vi "IO输出界面.vi"(8 "错误输入（无错误）":errorcluster, 10 "界面切换队列":refnum<queue>, 11 "VISA资源名称输入":refnum<visa-resource-name>) -> (0 "错误输出":errorcluster, 3 "VISA资源名称输出":refnum<visa-resource-name>)   [LabVIEW 2018]
panel:
  out "毫秒计时值":u32
  in  "枚举":T1(ring)
  in  "选项卡控件":enum32{"选项卡 1", "选项卡 2"}(tab)
  out "无":bool
  out "无":bool
  out "无":bool
  out "无":bool
  out "无":bool
  out "无":bool
  out "Y30D-11#启动":bool
  out "Y30E-13#启动":bool
  out "Y30F-15#启动":bool
  out "Y100-2#启动":bool
  out "Y101-4#启动":bool
  out "Y102-6#启动":bool
  out "Y103-8#启动":bool
  out "Y104-10#启动":bool
  out "Y105-12#启动":bool
  out "Y106-14#启动":bool
  out "Y107-16#启动":bool
  out "无":bool
  out "无":bool
  out "Y300-1#烧录气缸":bool
  out "Y301-2#烧录气缸":bool
  out "Y302-3#烧录气缸":bool
  out "Y303-4#烧录气缸":bool
  out "Y304-5#烧录气缸":bool
  out "Y305-6#烧录气缸":bool
  out "Y306-7#烧录气缸":bool
  out "Y307-8#烧录气缸":bool
  out "Y308-1#启动":bool
  out "Y309-3#启动":bool
  out "Y30A-5#启动":bool
  out "Y30B-7#启动":bool
  out "Y30C-9#启动":bool
  out "Y1A-蜂鸣器":bool
  out "Y1B-1号吸嘴真空":bool
  out "Y1C-2号吸嘴真空":bool
  out "Y1D-伺服报警清除":bool
  out "Y1E+空":bool
  out "Y1F-空":bool
  out "YD-自动换盘信号":bool
  out "YE-空":bool
  out "YF-空":bool
  out "Y10-启动灯":bool
  out "Y11-报警灯":bool
  out "Y12-停止灯":bool
  out "Y13-真空泵":bool
  out "Y14-1号吸嘴吹气":bool
  out "Y15":bool
  out "Y16-2号吸嘴吹气":bool
  out "Y17":bool
  out "Y18-1#飞达进料":bool
  out "Y19-2#飞达进料":bool
  out "DDT90356":dbl
  out "DDT90348":dbl
  out "自动界面":bool
  out "手动界面":bool
  out "参数界面":bool
  out "IO界面":bool
  out "产品界面":bool
  out "字符串":string
  out "DDT90352":dbl
  out "DDT90360":dbl
  out "DT1184":T2(ring)
  out "?":bool
  out "?":bool
  out "Y0-X轴脉冲":bool
  out "Y1-X轴方向":bool
  out "Y2-Y轴脉冲":bool
  out "Y3-Y轴方向":bool
  out "Y4-Z1轴脉冲":bool
  out "Y5-Z1轴方向":bool
  out "Y6-Z轴脉冲":bool
  out "Y7-Z轴方向":bool
  out "Y8-R1轴脉冲":bool
  out "Y9-R1轴方向":bool
  out "YA-R2轴脉冲":bool
  out "YB-R2轴方向":bool
  out "YC-卷带收料信号":bool
  out "通讯周期":dbl
  # "X"
  # "Z1"
  # "XXXXX自动化设备有限公司"
  # "Z2"
  # "Y"
  # "本\n体\n输\n出"
  # "扩\n展\n输\n出"
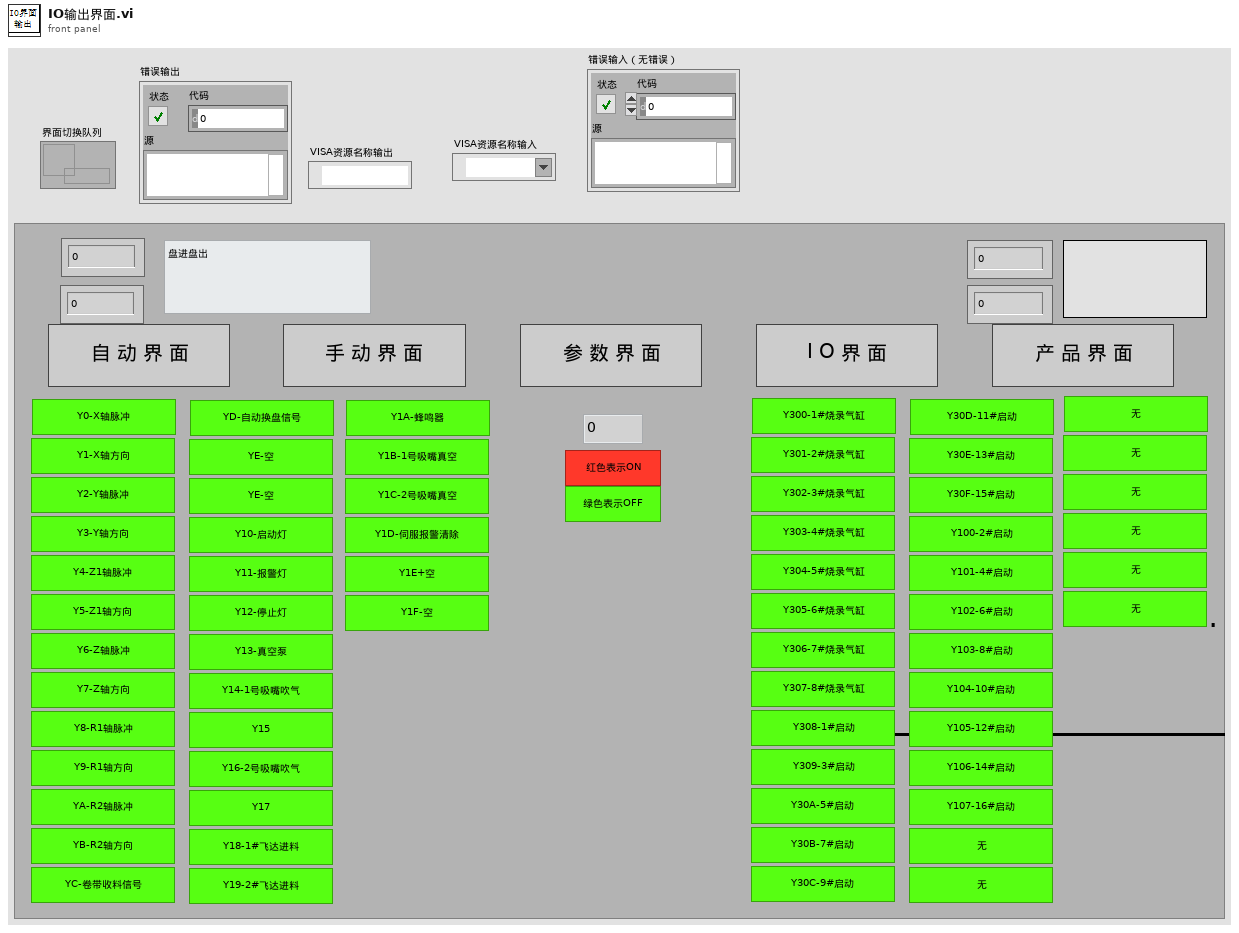
[diagram p1: front panel]
types:
  T1 = enum16{"读初始化", "读Y100+8", "读Y308+8", "读Y300+8", "读Y18+8", "读Y10+8", "读Y8-8", "读Y0+8", "读DDT90356", "读DT1184", "读DDT90348", ""}
  T2 = enum16{"盘进盘出", "卷进卷出", "盘进卷出", "管进盘出", "管进卷出", "卷进盘出", ""}
  T3 = enum8{"Enabled", "Disabled", "Disabled and Grayed Out"}
  T4 = typedef "数据簇.ctl" = cluster{"字符串":string, "数值":i32, "布尔":bool}
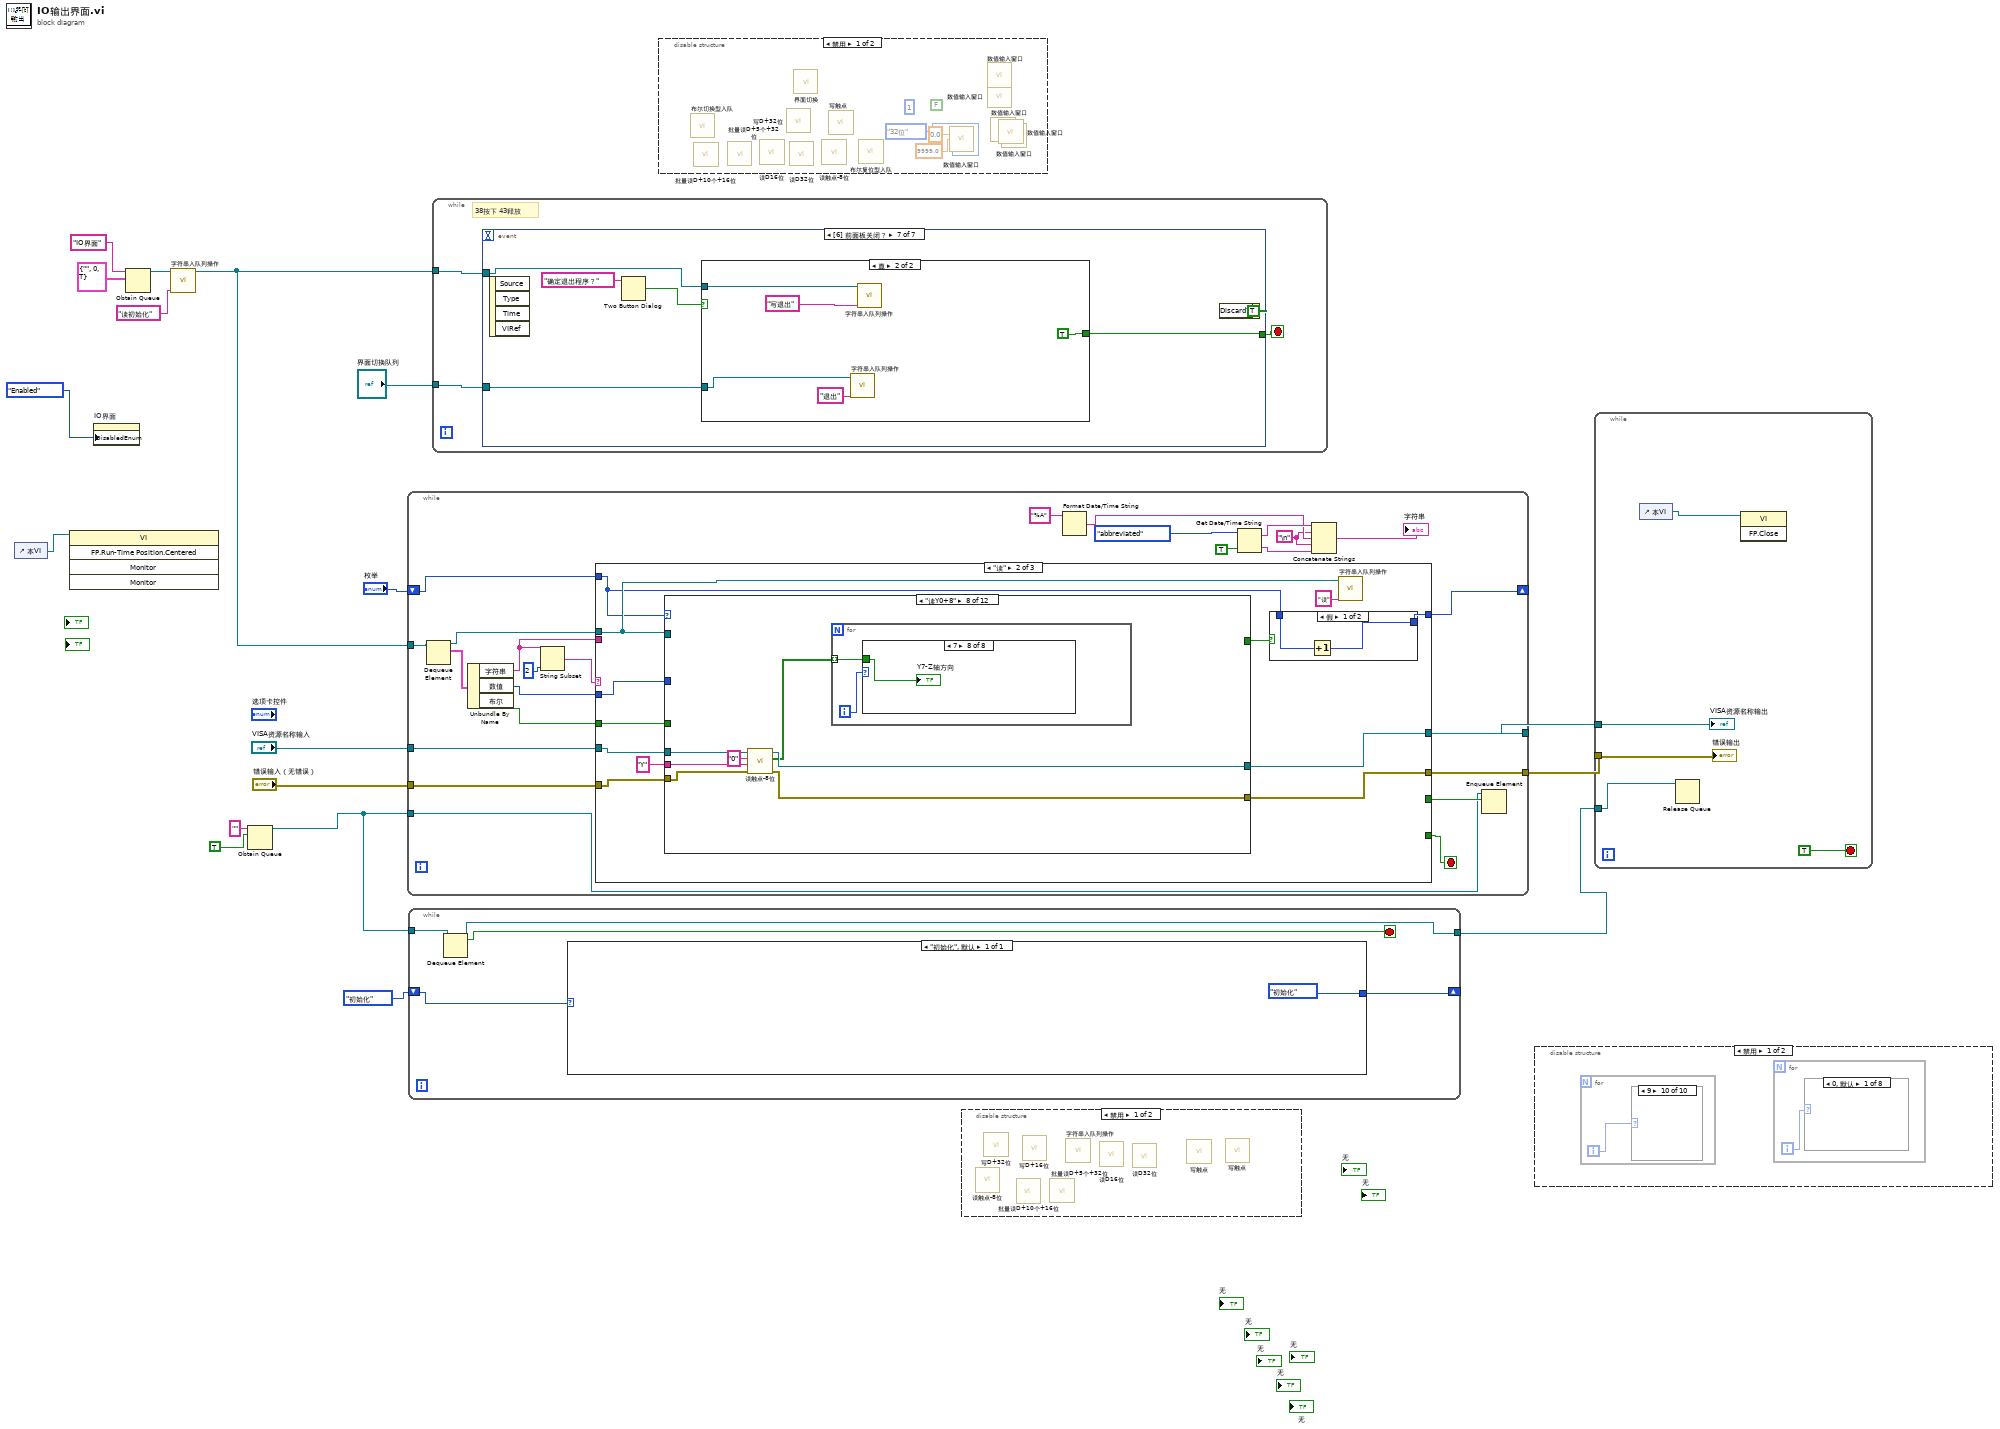
[diagram p0: block diagram]
diagram:
  n1 = control-ref of="本VI"() -> (w1:refnum<vi>)
  n2 = invoke class="VI" method="FP.Run-Time Position.Centered"(reference=w1) -> ()  [unwired: 4 in, 5 out]
  n3 = property on="IO界面" class="Bool"("DisabledEnum"=T3."Enabled" ("禁用")) -> ()  [unwired: 2 in, 2 out]
  n4 = Obtain Queue(name (unnamed)="IO界面" ("名称（未命名）"), element data type=T4 {"字符串"="", "数值"=0, "布尔"=TRUE}) -> (queue out=w11:refnum<queue>)  [unwired: 3 in, 2 out]
  n5 = call "字符串入队列操作.vi"("字符消息入队列"="读初始化", "界面切换队列"=w11) -> ("队列输出"=w3:refnum<queue>)  [unwired: 9 in]
  n6 = Obtain Queue(name (unnamed)="" ("名称（未命名）"), element data type=TRUE) -> (queue out=w6:refnum<queue>)  [unwired: 3 in, 2 out]
  n7 = while {
    tunnel: w3 -> [w39]
    tunnel: "VISA资源名称输入" -> [w32]
    tunnel: "错误输入（无错误）" -> [w31]
    tunnel: [w30] -> w13
    tunnel: [w29] -> w12
    shift-right: [w26] -> _
    shift-left: "枚举" -> [w27]
    tunnel: w6 -> [w19]
    stop <- w21 stop-if-true
    w23 = "\n"
    n8 = Dequeue Element(queue=w39) -> (queue out=w36:refnum<queue>, element=w38:T4)  [unwired: 2 in, 2 out]
    n9 = Unbundle By Name(w38) -> ("字符串"=w33:string, "数值"=w35:i32, "布尔"=w34:bool)
    n10 = String Subset(string=w33, length (rest)=2 ("长度（剩余）")) -> (substring=w37:string)  [unwired: 1 in]
    n11 = case shown="\"读\"" w37 {
      selector: w37 -> [w46 _ _]
      tunnel: w36 -> [_ w55 w243]
      tunnel: w35 -> [_ w62 w242]
      tunnel: w34 -> [_ w61 w241]
      tunnel: w33 -> [_ _ w235]
      tunnel: w32 -> [w45 w60 w240]
      tunnel: w31 -> [w44 w59 w239]
      tunnel: [w45 w58 w237] -> w30
      tunnel: [w44 w57 w236] -> w29
      tunnel: [_ _ w238] -> w21
      tunnel: w27 -> [_ w53 _]
      tunnel: [_ w52 _] -> w26
      tunnel: [_ _ w233] -> w20
      frame "", Default {
        n12 = Concatenate Strings("无对应消息分支**" ("消息"), w46, "**" ("字符串"), "读写状态机" ("字符串")) -> (w48:string)
        n13 = One Button Dialog(message=w48) -> ()  [unwired: 1 in, 1 out]
      }
      frame "读" {
        n14 = case shown="\"读Y0+8\"" w53 {
          tunnel: w55 -> [_ _ _ _ _ _ _ _ _ _ _ _]
          tunnel: w62 -> [_ _ _ _ _ _ _ _ _ _ _ _]
          tunnel: w60 -> [w67 w74 w91 w108 w125 w142 w159 w176 w198 w207 w220 w232]
          tunnel: w59 -> [w66 w73 w90 w106 w124 w141 w158 w175 w197 w206 w219 w231]
          tunnel: [w67 w72 w87 w104 w121 w140 w155 w172 w196 w205 w218 w232] -> w58
          tunnel: [w66 w71 w86 w103 w120 w139 w154 w171 w195 w204 w217 w231] -> w57
          tunnel: w61 -> [_ _ _ _ _ _ _ _ _ _ _ _]
          tunnel: [_ _ _ _ _ _ _ _ _ _ _ TRUE] -> w54
          tunnel: "Y" -> [_ w69 w88 w107 w123 w138 w157 w174 _ _ _ _]
          frame "读初始化" {
            n15 = Tick Count (ms)() -> (millisecond timer value=→"毫秒计时值":u32)
          }
          frame "读Y100+8" {
            n16 = call "读触点-8位.vi"("error out"=w73, "触点类型"=w69, "读取起始地址"="100", "VISA resource name out"=w74) -> ("error IO"=w71:errorcluster, "读取布尔数组"=w68:bool[], "VISA resource name out 2"=w72:refnum<visa-resource-name>)  [unwired: 4 in, 1 out]
            n17 = for {
              tunnel: w68 -> [w75] mode=indexing
              i -> [w76]
              n18 = case shown="7" w76 {
                tunnel: w75 -> [w77 w78 w79 w80 w81 w82 w83 w84]
                frame 0, Default {
                  "Y100-2#启动" <- w77
                }
                frame 1 {
                  "Y101-4#启动" <- w78
                }
                frame 2 {
                  "Y102-6#启动" <- w79
                }
                frame 3 {
                  "Y103-8#启动" <- w80
                }
                frame 4 {
                  "Y104-10#启动" <- w81
                }
                frame 5 {
                  "Y105-12#启动" <- w82
                }
                frame 6 {
                  "Y106-14#启动" <- w83
                }
                frame 7 {
                  "Y107-16#启动" <- w84
                }
              }
            }
          }
          frame "读Y308+8" {
            n19 = call "读触点-8位.vi"("error out"=w90, "触点类型"=w88, "读取起始地址"="308", "VISA resource name out"=w91) -> ("error IO"=w86:errorcluster, "读取布尔数组"=w85:bool[], "VISA resource name out 2"=w87:refnum<visa-resource-name>)  [unwired: 4 in, 1 out]
            n20 = for {
              tunnel: w85 -> [w92] mode=indexing
              i -> [w93]
              n21 = case shown="7" w93 {
                tunnel: w92 -> [w94 w95 w96 w97 w98 w99 w100 w101]
                frame 0, Default {
                  "Y308-1#启动" <- w94
                }
                frame 1 {
                  "Y309-3#启动" <- w95
                }
                frame 2 {
                  "Y30A-5#启动" <- w96
                }
                frame 3 {
                  "Y30B-7#启动" <- w97
                }
                frame 4 {
                  "Y30C-9#启动" <- w98
                }
                frame 5 {
                  "Y30D-11#启动" <- w99
                }
                frame 6 {
                  "Y30E-13#启动" <- w100
                }
                frame 7 {
                  "Y30F-15#启动" <- w101
                }
              }
            }
          }
          frame "读Y300+8" {
            n22 = call "读触点-8位.vi"("error out"=w106, "触点类型"=w107, "读取起始地址"="300", "VISA resource name out"=w108) -> ("error IO"=w103:errorcluster, "读取布尔数组"=w102:bool[], "VISA resource name out 2"=w104:refnum<visa-resource-name>)  [unwired: 4 in, 1 out]
            n23 = for {
              tunnel: w102 -> [w109] mode=indexing
              i -> [w110]
              n24 = case shown="7" w110 {
                tunnel: w109 -> [w111 w112 w113 w114 w115 w116 w117 w118]
                frame 0, Default {
                  "Y300-1#烧录气缸" <- w111
                }
                frame 1 {
                  "Y301-2#烧录气缸" <- w112
                }
                frame 2 {
                  "Y302-3#烧录气缸" <- w113
                }
                frame 3 {
                  "Y303-4#烧录气缸" <- w114
                }
                frame 4 {
                  "Y304-5#烧录气缸" <- w115
                }
                frame 5 {
                  "Y305-6#烧录气缸" <- w116
                }
                frame 6 {
                  "Y306-7#烧录气缸" <- w117
                }
                frame 7 {
                  "Y307-8#烧录气缸" <- w118
                }
              }
            }
          }
          frame "读Y18+8" {
            n25 = call "读触点-8位.vi"("error out"=w124, "触点类型"=w123, "读取起始地址"="18", "VISA resource name out"=w125) -> ("error IO"=w120:errorcluster, "读取布尔数组"=w119:bool[], "VISA resource name out 2"=w121:refnum<visa-resource-name>)  [unwired: 4 in, 1 out]
            n26 = for {
              tunnel: w119 -> [w126] mode=indexing
              i -> [w127]
              n27 = case shown="1" w127 {
                tunnel: w126 -> [w128 w129 w130 w131 w132 w133 w134 w135]
                frame 0, Default {
                  "Y18-1#飞达进料" <- w128
                }
                frame 1 {
                  "Y19-2#飞达进料" <- w129
                }
                frame 2 {
                  "Y1A-蜂鸣器" <- w130
                }
                frame 3 {
                  "Y1B-1号吸嘴真空" <- w131
                }
                frame 4 {
                  "Y1C-2号吸嘴真空" <- w132
                }
                frame 5 {
                  "Y1D-伺服报警清除" <- w133
                }
                frame 6 {
                  "Y1E+空" <- w134
                }
                frame 7 {
                  "Y1F-空" <- w135
                }
              }
            }
          }
          frame "读Y10+8" {
            n28 = call "读触点-8位.vi"("error out"=w141, "触点类型"=w138, "读取起始地址"="10", "VISA resource name out"=w142) -> ("error IO"=w139:errorcluster, "读取布尔数组"=w136:bool[], "VISA resource name out 2"=w140:refnum<visa-resource-name>)  [unwired: 4 in, 1 out]
            n29 = for {
              tunnel: w136 -> [w143] mode=indexing
              i -> [w144]
              n30 = case shown="7" w144 {
                tunnel: w143 -> [w145 w146 w147 w148 w149 w150 w151 w152]
                frame 0, Default {
                  "Y10-启动灯" <- w145
                }
                frame 1 {
                  "Y11-报警灯" <- w146
                }
                frame 2 {
                  "Y12-停止灯" <- w147
                }
                frame 3 {
                  "Y13-真空泵" <- w148
                }
                frame 4 {
                  "Y14-1号吸嘴吹气" <- w149
                }
                frame 5 {
                  "Y15" <- w150
                }
                frame 6 {
                  "Y16-2号吸嘴吹气" <- w151
                }
                frame 7 {
                  "Y17" <- w152
                }
              }
            }
          }
          frame "读Y8-8" {
            n31 = call "读触点-8位.vi"("error out"=w158, "触点类型"=w157, "读取起始地址"="8", "VISA resource name out"=w159) -> ("error IO"=w154:errorcluster, "读取布尔数组"=w153:bool[], "VISA resource name out 2"=w155:refnum<visa-resource-name>)  [unwired: 4 in, 1 out]
            n32 = for {
              tunnel: w153 -> [w160] mode=indexing
              i -> [w161]
              n33 = case shown="7" w161 {
                tunnel: w160 -> [w162 w163 w164 w165 w166 w167 w168 w169]
                frame 0, Default {
                  "Y8-R1轴脉冲" <- w162
                }
                frame 1 {
                  "Y9-R1轴方向" <- w163
                }
                frame 2 {
                  "YA-R2轴脉冲" <- w164
                }
                frame 3 {
                  "YB-R2轴方向" <- w165
                }
                frame 4 {
                  "YC-卷带收料信号" <- w166
                }
                frame 5 {
                  "YD-自动换盘信号" <- w167
                }
                frame 6 {
                  "YE-空" <- w168
                }
                frame 7 {
                  "YF-空" <- w169
                }
              }
            }
          }
          frame "读Y0+8" {
            n34 = call "读触点-8位.vi"("error out"=w175, "触点类型"=w174, "读取起始地址"="0", "VISA resource name out"=w176) -> ("error IO"=w171:errorcluster, "读取布尔数组"=w170:bool[], "VISA resource name out 2"=w172:refnum<visa-resource-name>)  [unwired: 4 in, 1 out]
            n35 = for {
              tunnel: w170 -> [w177] mode=indexing
              i -> [w178]
              n36 = case shown="7" w178 {
                tunnel: w177 -> [w179 w180 w181 w182 w183 w184 w185 w186]
                frame 0, Default {
                  "Y0-X轴脉冲" <- w179
                }
                frame 1 {
                  "Y1-X轴方向" <- w180
                }
                frame 2 {
                  "Y2-Y轴脉冲" <- w181
                }
                frame 3 {
                  "Y3-Y轴方向" <- w182
                }
                frame 4 {
                  "Y4-Z1轴脉冲" <- w183
                }
                frame 5 {
                  "Y5-Z1轴方向" <- w184
                }
                frame 6 {
                  "Y6-Z轴脉冲" <- w185
                }
                frame 7 {
                  "Y7-Z轴方向" <- w186
                }
              }
            }
          }
          frame "读DDT90356" {
            n37 = call "批量读D+5个+32位.vi"("error out"=w197, "读取D地址"=90356, "VISA resource name out"=w198) -> ("error IO"=w195:errorcluster, "数组"=w201:i32[], "VISA resource name out 2"=w196:refnum<visa-resource-name>)  [unwired: 5 in, 1 out]
            n38 = Index Array(array=w201, index #1=0 ("索引"), index #2=2 ("索引")) -> (element #1=w194:i32, element #2=w193:i32)
            n39 = To Double Precision Float(number=w194) -> (double precision float=w192:dbl)
            n40 = To Double Precision Float(number=w193) -> (double precision float=w189:dbl)
            n41 = Divide(x=w192, y=100.0) -> (x/y=→"DDT90356":dbl)
            n42 = Divide(x=w189, y=100.0) -> (x/y=→"DDT90360":dbl)
          }
          frame "读DT1184" {
            n43 = call "读D16位.vi"("error out"=w206, "读取D地址"=1184, "VISA resource name out"=w207) -> ("error IO"=w204:errorcluster, "数值"=→"DT1184":u32, "VISA resource name out 2"=w205:refnum<visa-resource-name>)  [unwired: 5 in, 1 out]
          }
          frame "读DDT90348" {
            n44 = call "批量读D+5个+32位.vi"("error out"=w219, "读取D地址"=90348, "VISA resource name out"=w220) -> ("error IO"=w217:errorcluster, "数组"=w224:i32[], "VISA resource name out 2"=w218:refnum<visa-resource-name>)  [unwired: 5 in, 1 out]
            n45 = Index Array(array=w224, index #1=0 ("索引"), index #2=2 ("索引")) -> (element #1=w216:i32, element #2=w215:i32)
            n46 = To Double Precision Float(number=w215) -> (double precision float=w210:dbl)
            n47 = To Double Precision Float(number=w216) -> (double precision float=w214:dbl)
            n48 = Divide(x=w210, y=100.0) -> (x/y=→"DDT90352":dbl)
            n49 = Divide(x=w214, y=100.0) -> (x/y=→"DDT90348":dbl)
          }
          frame "" {
            n50 = local read "毫秒计时值"() -> (w228:u32)
            n51 = Tick Count (ms)() -> (millisecond timer value=w229:u32)
            n52 = Subtract(x=w229, y=w228) -> (x-y=w227:u32)
            n53 = Divide(x=w227, y=u32 1000) -> (x/y=→"通讯周期":dbl)
          }
        }
        n54 = case shown="假" w54 {
          tunnel: w53 -> [w64 _]
          tunnel: [w63 _] -> w52
          frame False {
            n55 = Increment(x=w64) -> (x+1=w63:T1)
          }
          frame True {
          }
        }
        n56 = call "字符串入队列操作.vi"("字符消息入队列"="读", "界面切换队列"=w55) -> ()  [unwired: 9 in, 1 out]
      }
      frame "写" {
        n57 = call "状态匹配.vi"("输入状态"=w235) -> ("输出状态"=w234:string)  [unwired: 10 in]
        n58 = case shown="\"写R\"" w234 {
          selector: w234 -> [w246 _ _ _ _]
          tunnel: w243 -> [_ _ _ _ w286]
          tunnel: w242 -> [_ w252 w269 _ _]
          tunnel: w241 -> [_ _ _ w280 _]
          tunnel: w240 -> [w245 w262 w273 w285 w291]
          tunnel: w239 -> [w244 w261 w272 w284 w290]
          tunnel: [_ _ _ _ w289] -> w238
          tunnel: [w245 w260 w271 w283 w291] -> w237
          tunnel: [w244 w259 w270 w282 w290] -> w236
          tunnel: w235 -> [_ w251 w263 w274 _]
          tunnel: [_ _ _ _ w289] -> w233
          frame "", Default {
            n59 = Concatenate Strings("无对应消息分支**" ("消息"), w246, "**" ("字符串"), "写状态机" ("字符串")) -> (w250:string)
            n60 = One Button Dialog(message=w250) -> ()  [unwired: 1 in, 1 out]
          }
          frame "写DT" {
            n61 = String Length(string=w251) -> (length=w257:i32)
            n62 = Subtract(x=w257, y=4) -> (x-y=w255:i32)
            n63 = String Subset(string=w251, offset (0)=4 ("偏移量(0)"), length (rest)=w255) -> (substring=w254:string)
            n64 = Decimal String To Number(string=w254) -> (number=w253:i32)  [unwired: 2 in, 1 out]
            n65 = call "写D+16位.vi"("error out"=w261, "输入数值"=w252, "输入地址D"=w253, "VISA resource name out"=w262) -> ("error out 2"=w259:errorcluster, "VISA resource name out 2"=w260:refnum<visa-resource-name>)  [unwired: 3 in, 3 out]
          }
          frame "写DDT" {
            n66 = String Length(string=w263) -> (length=w267:i32)
            n67 = Subtract(x=w267, y=5) -> ()  [unwired: 1 out]
            n68 = String Subset(string=w263, offset (0)=5 ("偏移量(0)")) -> (substring=w264:string)  [unwired: 1 in]
            n69 = Decimal String To Number(string=w264) -> (number=w265:i32)  [unwired: 2 in, 1 out]
            n70 = call "写D+32位.vi"("error out"=w272, "输入数值"=w269, "输入地址D"=w265, "VISA resource name out"=w273) -> ("error out 2"=w270:errorcluster, "VISA resource name out 2"=w271:refnum<visa-resource-name>)  [unwired: 4 in, 2 out]
          }
          frame "写R" {
            n71 = String Length(string=w274) -> (length=w278:i32)
            n72 = Subtract(x=w278, y=3) -> (x-y=w276:i32)
            n73 = String Subset(string=w274, offset (0)=3 ("偏移量(0)"), length (rest)=w276) -> (substring=w275:string)
            n74 = call "写触点.vi"("布尔"=w280, "error out"=w284, "触点类型"="R", "写入起始地址"=w275, "VISA resource name out"=w285) -> ("error IO"=w282:errorcluster, "VISA resource name out 2"=w283:refnum<visa-resource-name>)  [unwired: 4 in, 1 out]
          }
          frame "写退出" {
            w289 = TRUE
            n75 = Flush Queue(queue=w286) -> (queue out=w287:refnum<queue>, error out=w288:errorcluster)  [unwired: 1 in, 1 out]
            n76 = Release Queue(queue=w287, error in (no error)=w288) -> ()  [unwired: 1 in, 3 out]
          }
        }
      }
    }
    n77 = Format Date/Time String(time format string (%c)="%A" ("时间格式字符串(%c)")) -> (date/time string=w24:string)  [unwired: 2 in]
    n78 = Get Date/Time String(date format (0)=enum16{"short", "long", "abbreviated"}."abbreviated" ("日期格式(0)"), want seconds? (F)=TRUE ("需要秒？(F)")) -> (date string=w41:string, time string=w22:string)  [unwired: 1 in]
    n79 = Concatenate Strings(w41, w23, w24, w23, w22) -> (→"字符串":string)
    n80 = Enqueue Element(queue=w19, element=w20) -> ()  [unwired: 2 in, 3 out]
  }
  n81 = while {
    shift-right: [w295] -> _
    shift-left: enum16{"初始化"}."初始化" -> [w296]
    tunnel: w6 -> [w294]
    tunnel: [w292] -> w5
    stop <- w293 stop-if-true
    n82 = Dequeue Element(queue=w294) -> (queue out=w292:refnum<queue>, element=w293:bool)  [unwired: 2 in, 2 out]
    n83 = case shown="\"初始化\", 默认" w296 {
      tunnel: [enum16{"初始化"}."初始化"] -> w295
      frame "初始化", Default {
      }
    }
  }
  n84 = while {
    tunnel: w3 -> [w300]
    tunnel: "界面切换队列" -> [w299]
    stop <- w298 stop-if-true
    # "38按下 43释放"
    n85 = event shown="[6] 前面板关闭？" {
      selector: _ -> [_ _ _ _ _ _ _]
      dyn-events: _ -> [_ _ _ _ _ _ _]
      timeout: _ -> [_ _ _ _ _ _ _]
      tunnel: w300 -> [w305 w310 w315 w320 w324 _ w327]
      tunnel: w299 -> [w304 w308 w314 w319 w323 _ w326]
      tunnel: [w301 w309 w311 w316 _ _ w325] -> w298
      event "IO界面": Mouse Down {
        n86 = event-data() -> ("CtlRef"=w303:refnum<vi>)  [unwired: 1 in, 7 out]
        n87 = call "界面切换.vi"("界面切换队列输入"=w304, "切换界面名称输入"="IO界面", "Bool引用句柄"=w303, "状态转移输入"=w305) -> ("布尔"=w301:bool)  [unwired: 7 in]
      }
      event "参数界面": Mouse Down {
        n88 = event-data() -> ("CtlRef"=w307:refnum<vi>)  [unwired: 1 in, 7 out]
        n89 = call "界面切换.vi"("界面切换队列输入"=w308, "切换界面名称输入"="参数界面", "Bool引用句柄"=w307, "状态转移输入"=w310) -> ("布尔"=w309:bool)  [unwired: 7 in]
      }
      event "产品界面": Mouse Down {
        n90 = event-data() -> ("CtlRef"=w313:refnum<vi>)  [unwired: 1 in, 7 out]
        n91 = call "界面切换.vi"("界面切换队列输入"=w314, "切换界面名称输入"="产品界面", "Bool引用句柄"=w313, "状态转移输入"=w315) -> ("布尔"=w311:bool)  [unwired: 7 in]
      }
      event "手动界面": Mouse Down {
        n92 = event-data() -> ("CtlRef"=w318:refnum<vi>)  [unwired: 1 in, 7 out]
        n93 = call "界面切换.vi"("界面切换队列输入"=w319, "切换界面名称输入"="手动界面", "Bool引用句柄"=w318, "状态转移输入"=w320) -> ("布尔"=w316:bool)  [unwired: 7 in]
      }
      event "自动界面": Mouse Down {
        n94 = event-data() -> ("CtlRef"=w321:refnum<vi>)  [unwired: 1 in, 7 out]
        n95 = call "界面切换.vi"("界面切换队列输入"=w323, "切换界面名称输入"="自动界面", "Bool引用句柄"=w321, "状态转移输入"=w324) -> ()  [unwired: 7 in, 1 out]
      }
      event Timeout {
        n96 = event-data() -> ()  [unwired: 1 in, 3 out]
      }
      event Panel Close? {
        n97 = event-data() -> ()  [unwired: 1 in, 4 out]
        n98 = Two Button Dialog(message="确定退出程序？" ("消息")) -> (T button?=w328:bool)  [unwired: 2 in]
        n99 = case shown="真" w328 {
          tunnel: [_ TRUE] -> w325
          tunnel: w327 -> [_ w333]
          tunnel: w326 -> [_ w332]
          frame False {
          }
          frame True {
            n100 = call "字符串入队列操作.vi"("字符消息入队列"="退出", "界面切换队列"=w332) -> ()  [unwired: 9 in, 1 out]
            n101 = call "字符串入队列操作.vi"("字符消息入队列"="写退出", "界面切换队列"=w333) -> ()  [unwired: 9 in, 1 out]
          }
        }
        n102 = event-data("Discard?"=TRUE ("放弃？")) -> ()  [unwired: 1 in, 1 out]
      }
    }
  }
  n103 = disable-structure shown="禁用" {
    frame Disabled {
      (unwired) u32 1 ("转换比例")
      (unwired) FALSE ("忽略数值上下限")
      n104 = call "布尔切换型入队.vi"() -> ()  [unwired: 12 in]
      n105 = call "批量读D+10个+16位.vi"() -> ()  [unwired: 8 in, 4 out]
      n106 = call "批量读D+5个+32位.vi"() -> ()  [unwired: 8 in, 4 out]
      n107 = call "读D16位.vi"() -> ()  [unwired: 8 in, 4 out]
      n108 = call "写D+32位.vi"() -> ()  [unwired: 8 in, 4 out]
      n109 = call "读D32位.vi"() -> ()  [unwired: 9 in, 3 out]
      n110 = call "界面切换.vi"() -> ()  [unwired: 11 in, 1 out]
      n111 = call "读触点-8位.vi"() -> ()  [unwired: 8 in, 4 out]
      n112 = call "写触点.vi"() -> ()  [unwired: 9 in, 3 out]
      n113 = call "布尔复位型入队.vi"() -> ()  [unwired: 8 in, 2 out]
      n114 = call "数值输入窗口.vi"("输入下限"=0.0, "输入上限"=9999.0, "数据类型"=enum16{"32位", "16位"}."32位") -> ("转换比例"=w339:u32)  [unwired: 9 in, 3 out]
      n115 = call "数值输入窗口.vi"() -> ()  [unwired: 13 in, 3 out]
      n116 = call "数值输入窗口.vi"() -> ()  [unwired: 13 in, 3 out]
      n117 = call "数值输入窗口.vi"() -> ()  [unwired: 13 in, 3 out]
      n118 = call "数值输入窗口.vi"() -> ()  [unwired: 13 in, 3 out]
      n119 = call "数值输入窗口.vi"() -> ()  [unwired: 13 in, 3 out]
    }
    frame Enabled {
    }
  }
  n120 = disable-structure shown="禁用" {
    frame Disabled {
      n121 = call "读触点-8位.vi"() -> ()  [unwired: 8 in, 4 out]
      n122 = call "写D+32位.vi"() -> ()  [unwired: 8 in, 4 out]
      n123 = call "批量读D+10个+16位.vi"() -> ()  [unwired: 8 in, 4 out]
      n124 = call "写D+16位.vi"() -> ()  [unwired: 7 in, 5 out]
      n125 = call "批量读D+5个+32位.vi"() -> ()  [unwired: 8 in, 4 out]
      n126 = call "字符串入队列操作.vi"() -> ()  [unwired: 11 in, 1 out]
      n127 = call "读D16位.vi"() -> ()  [unwired: 8 in, 4 out]
      n128 = call "读D32位.vi"() -> ()  [unwired: 9 in, 3 out]
      n129 = call "写触点.vi"() -> ()  [unwired: 9 in, 3 out]
      n130 = call "写触点.vi"() -> ()  [unwired: 9 in, 3 out]
    }
    frame Enabled {
    }
  }
  n131 = disable-structure shown="禁用" {
    frame Disabled {
      n132 = for {
        i -> [w341]
        n133 = case shown="9" w341 {
          frame 0, Default {
          }
          frame 1 {
          }
          frame 2 {
          }
          frame 3 {
          }
          frame 4 {
          }
          frame 5 {
          }
          frame 6 {
          }
          frame 7 {
          }
          frame 8 {
          }
          frame 9 {
          }
        }
      }
      n134 = for {
        i -> [w340]
        n135 = case shown="0, 默认" w340 {
          frame 0, Default {
          }
          frame 1 {
          }
          frame 2 {
          }
          frame 3 {
          }
          frame 4 {
          }
          frame 5 {
          }
          frame 6 {
          }
          frame 7 {
          }
        }
      }
    }
    frame Enabled {
    }
  }
  n136 = while {
    tunnel: w13 -> [w345]
    tunnel: w12 -> [w344]
    tunnel: w5 -> [w343]
    stop <- TRUE stop-if-true
    n137 = control-ref of="本VI"() -> (w342:refnum<vi>)
    n138 = Release Queue(queue=w343) -> ()  [unwired: 2 in, 3 out]
    n139 = invoke class="VI" method="FP.Close"(reference=w342) -> ()  [unwired: 2 in, 3 out]
    "VISA资源名称输出" <- w345
    "错误输出" <- w344
  }
